vi "Close.vi"(0 "SLSC Remote in":refnum<class "SLSC Remote.lvclass">, 11 "error in (no error)":errorcluster) -> (15 "error out":errorcluster)   [LabVIEW 2015, in "SLSC Remote.lvclass"]
uses:
  SLSC Remote.lvclass
  <vilib>/NI/i3 JSON/JSON Generation/Create Value Files/Create Value - Object.vi
  <vilib>/NI/i3 JSON/JSON Generation/Add Object Parameter Files/Add Object Parameter - String.vi
  <vilib>/NI/NI JSONRPC Server Framework/Classes/Server/Format Client Request (Auto-Increment).vi
  <vilib>/httpClient/POSTBuffer.vi
  <vilib>/NI/NI JSONRPC Server Framework/Classes/Server/JSONRPC Server.lvclass
  <vilib>/NI/i3 JSON/i3-json.lvlib
  <vilib>/httpClient/LabVIEWHTTPClient.lvlib
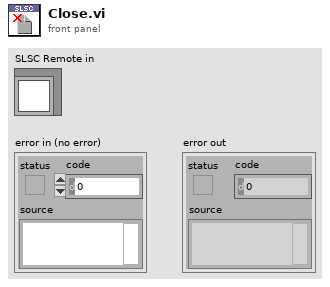
[diagram p1: front panel]
types:
  T1 = typedef "LabVIEWHTTPClient.lvlib/ClientHandle.ctl" = refnum<k1>
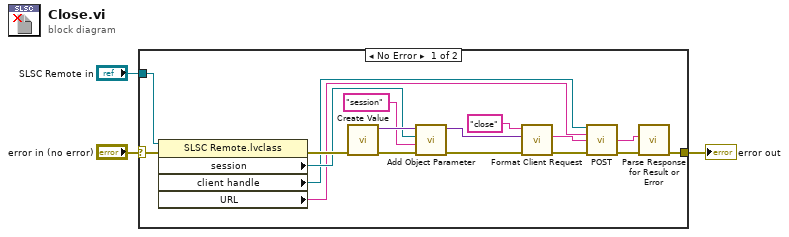
[diagram p0: block diagram]
diagram:
  n1 = case shown="No Error" "error in (no error)" {
    selector: "error in (no error)" -> [w18 w21]
    tunnel: "SLSC Remote in" -> [w19 _]
    tunnel: [w4 w21] -> w1
    frame No Error {
      n2 = property class="SLSC Remote.lvclass"(reference=w19, error in=w18) -> (error out=w17:errorcluster, "session"=w13:refnum<k21>, "client handle"=w9:T1, "URL"=w8:string)  [unwired: 1 out]
      n3 = call-poly <vilib>:"Create Value.vi"("error in (no error)"=w17) -> ("error out"=w16:errorcluster, "JSON Tree"=w20:variant)  [unwired: 9 in]
      n4 = call-poly <vilib>:"Add Object Parameter.vi"("error in (no error)"=w16, "Name"="session", "String"=w13, "JSON Tree in (JSON Object)"=w20) -> ("error out"=w10:errorcluster, "JSON Tree out (JSON Object)"=w11:variant)  [unwired: 6 in]
      n5 = call-poly <vilib>:"Format Client Request.vi"("error in (no error)"=w10, "params"=w11, "method"="close") -> ("error out"=w7:errorcluster, "Request String"=w14:string)  [unwired: 7 in]
      n6 = call-poly <vilib>:"POST.vi"("client handle"=w9, "url"=w8, "buffer"=w14, "error in (no error)"=w7) -> ("body"=w6:string, "error out"=w5:errorcluster)  [unwired: 8 in, 2 out]
      n7 = call <vilib>:"Parse Response for Result or Error.vi"("error in"=w5, "Response String In"=w6) -> ("error out"=w4:errorcluster)  [unwired: 7 in, 2 out]
    }
    frame Error {
    }
  }
  "error out" <- w1
